vi "float_to_string.vi"(9 "Float format":T1, 10 "Float":dbl) -> (2 "String":string)   [LabVIEW 2018]
doc: "Format a float as an IC6 defined REAL_4X1 string."
uses:
  float_format_codes.ctl
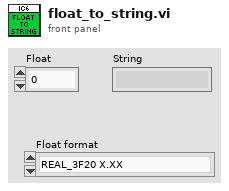
[diagram p1: front panel]
types:
  T1 = typedef "float_format_codes.ctl" = enum16{"REAL_3F20 X.XX", "REAL_3F20 XX.X", "REAL_3F20 XXX", "REAL_3X1", "REAL_4F21 XX.XX", "REAL_4F21 XXX.X", "REAL_4F31 X.XXX", "REAL_4F31 XX.XX", "REAL_4F31 XXX.X", "REAL_4X1", "REAL_4X2", "REAL_4X3", "REAL_5F32 XX.XXX", "REAL_5F32 XXX.XX", "REAL_5X2", "REAL_5X3", "REAL_6F32 XXX.XXX", "REAL_6F32 XXXX.XX"}
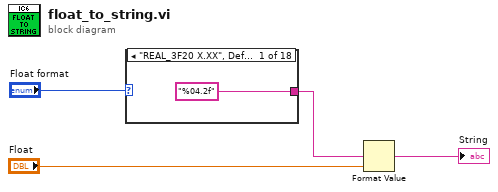
[diagram p0: block diagram]
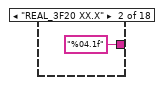
[diagram p2: hidden frame]
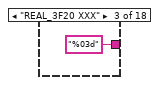
[diagram p3: hidden frame]
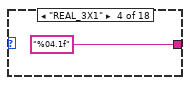
[diagram p4: hidden frame]
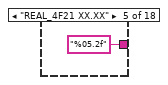
[diagram p5: hidden frame]
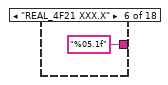
[diagram p6: hidden frame]
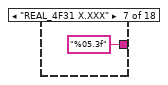
[diagram p7: hidden frame]
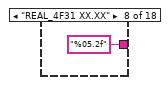
[diagram p8: hidden frame]
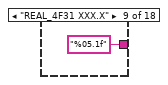
[diagram p9: hidden frame]
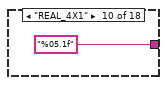
[diagram p10: hidden frame]
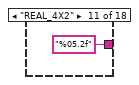
[diagram p11: hidden frame]
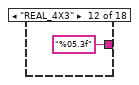
[diagram p12: hidden frame]
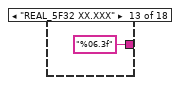
[diagram p13: hidden frame]
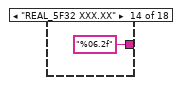
[diagram p14: hidden frame]
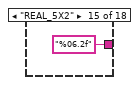
[diagram p15: hidden frame]
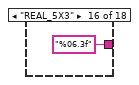
[diagram p16: hidden frame]
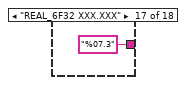
[diagram p17: hidden frame]
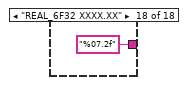
[diagram p18: hidden frame]
diagram:
  n1 = case shown="\"REAL_3F20 X.XX\", Default" "Float format" {
    tunnel: ["%04.2f" ("format string") "%04.1f" ("format string") "%03d" ("format string") "%04.1f" ("format string") "%05.2f" ("format string") "%05.1f" ("format string") "%05.3f" ("format string") "%05.2f" ("format string") "%05.1f" ("format string") "%05.1f" "%05.2f" ("format string") "%05.3f" ("format string") "%06.3f" ("format string") "%06.2f" ("format string") "%06.2f" ("format string") "%06.3f" ("format string") "%07.3" ("format string") "%07.2f" ("format string")] -> w1
    frame "REAL_3F20 X.XX", Default {
    }
    frame "REAL_3F20 XX.X" {
    }
    frame "REAL_3F20 XXX" {
    }
    frame "REAL_3X1" {
    }
    frame "REAL_4F21 XX.XX" {
    }
    frame "REAL_4F21 XXX.X" {
    }
    frame "REAL_4F31 X.XXX" {
    }
    frame "REAL_4F31 XX.XX" {
    }
    frame "REAL_4F31 XXX.X" {
    }
    frame "REAL_4X1" {
    }
    frame "REAL_4X2" {
    }
    frame "REAL_4X3" {
    }
    frame "REAL_5F32 XX.XXX" {
    }
    frame "REAL_5F32 XXX.XX" {
    }
    frame "REAL_5X2" {
    }
    frame "REAL_5X3" {
    }
    frame "REAL_6F32 XXX.XXX" {
    }
    frame "REAL_6F32 XXXX.XX" {
    }
  }
  n2 = Format Value(format string=w1, value (0)="Float") -> (output string=→"String":string)  [unwired: 1 in]
